vi "Check if Add States to Queue is Primary One.vi"(8 "error in (no error)":errorcluster, 11 "Add State(s) to Queue ref":refnum<vi>) -> (0 "error out":errorcluster, 2 "Is Primary?":bool)   [LabVIEW 2020, in "JKI State Machine API.lvlib" / "JKI SM.lvclass"]
uses:
  JKI SM.lvclass
  JKI SM.lvclass/JKI SM.ctl
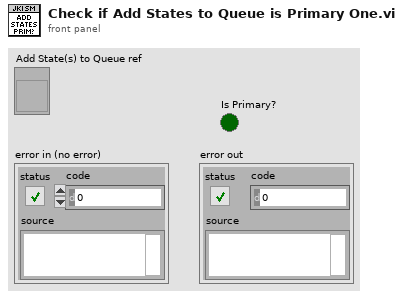
[diagram p1: front panel]
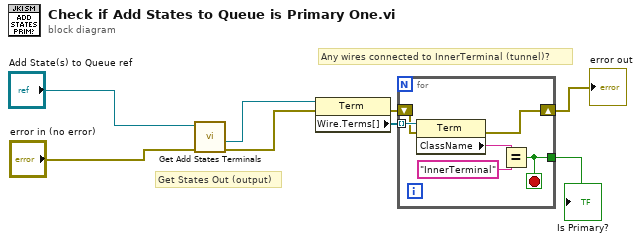
[diagram p0: block diagram]
diagram:
  # "Get States Out (output)"
  # "Any wires connected to InnerTerminal (tunnel)?"
  n1 = call "Get Add States Terminals.vi"("error in (no error)"="error in (no error)", "Add State(s) to Queue ref"="Add State(s) to Queue ref") -> ("error out"=w2:errorcluster, "States Out"=w1:refnum<vi>)  [unwired: 5 in, 3 out]
  n2 = property class="Term"(reference=w1, error in=w2) -> (error out=w7:errorcluster, "Wire.Terms[]"=w5:refnum<vi>[])  [unwired: 1 out]
  n3 = for {
    tunnel: w5 -> [w14] mode=indexing
    tunnel: [w11] -> w6
    shift-right: [w10] -> w8
    shift-left: w7 -> [w9]
    stop <- w11 stop-if-true
    n4 = property class="Term"(reference=w14, error in=w9) -> (error out=w10:errorcluster, "ClassName"=w12:string)  [unwired: 1 out]
    n5 = Equal?(x=w12, y="InnerTerminal" ("Class Name")) -> (x = y?=w11:bool)
  }
  "error out" <- w8
  "Is Primary?" <- w6
